vi "PicoScope4000aSetupStreaming.vi"(0 "error in":errorcluster, 2 "handle in":i16, 3 "Acquisition Settings":T2={"Auto Stop"=FALSE, "Desired Sample Interval"=4, "Pre-trigger Samples"=0, "Post-trigger Samples"=1000, "Down-Sample Ratio"=1, "Down-Sample Mode"=0, "Time Units"=2} {"Time Units" items=["Nanoseconds (ns)"=2, "Microseconds (us)"=3, "Milliseconds (ms)"=4, "Seconds (s)"=5]; "Down-Sample Mode" items=["None"=0, "Aggregate"=1, "Decimate"=2, "Average"=4]}, 4 "Buffer and Transfer Settings":T1={"startIndex"=0, "Samples"=1000000, "Down Sample Ratio"=1, "Down-Sample Mode"=0} {"Down-Sample Mode" items=["None"=0, "Aggregate"=1, "Decimate"=2, "Average"=4]; "Down Sample Ratio" step=1; "Samples" format="%_6p"}, 5 "enabled array":i16[](array[numeric]), 10 "Pointers In":u64[][](array[numeric])) -> (11 "Pointer array":u64[][](array[numeric]), 14 "error out":errorcluster, 16 "handle out":i16, 17 "Sample Interval":u32, 19 "sampleIntervalTimeUnits":u32)   [LabVIEW 2016]
doc: "Set up the data buffers and calls RunStreaming to start the device streaming.\nData will be copied from the driver buffers into the corresponding application buffers using the wrapper dll."
uses:
  ps4000a.dll
  ps4000aWrap.dll
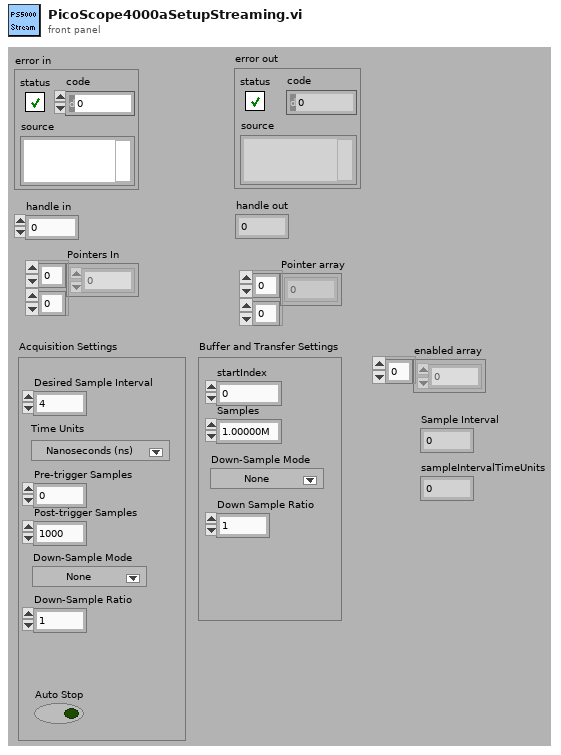
[diagram p1: front panel]
types:
  T1 = cluster{"startIndex":u64, "Samples":u64, "Down Sample Ratio":u64, "Down-Sample Mode":u32}
  T2 = cluster{"Auto Stop":bool, "Desired Sample Interval":u32, "Pre-trigger Samples":u32, "Post-trigger Samples":u32, "Down-Sample Ratio":u32, "Down-Sample Mode":i32, "Time Units":u32}
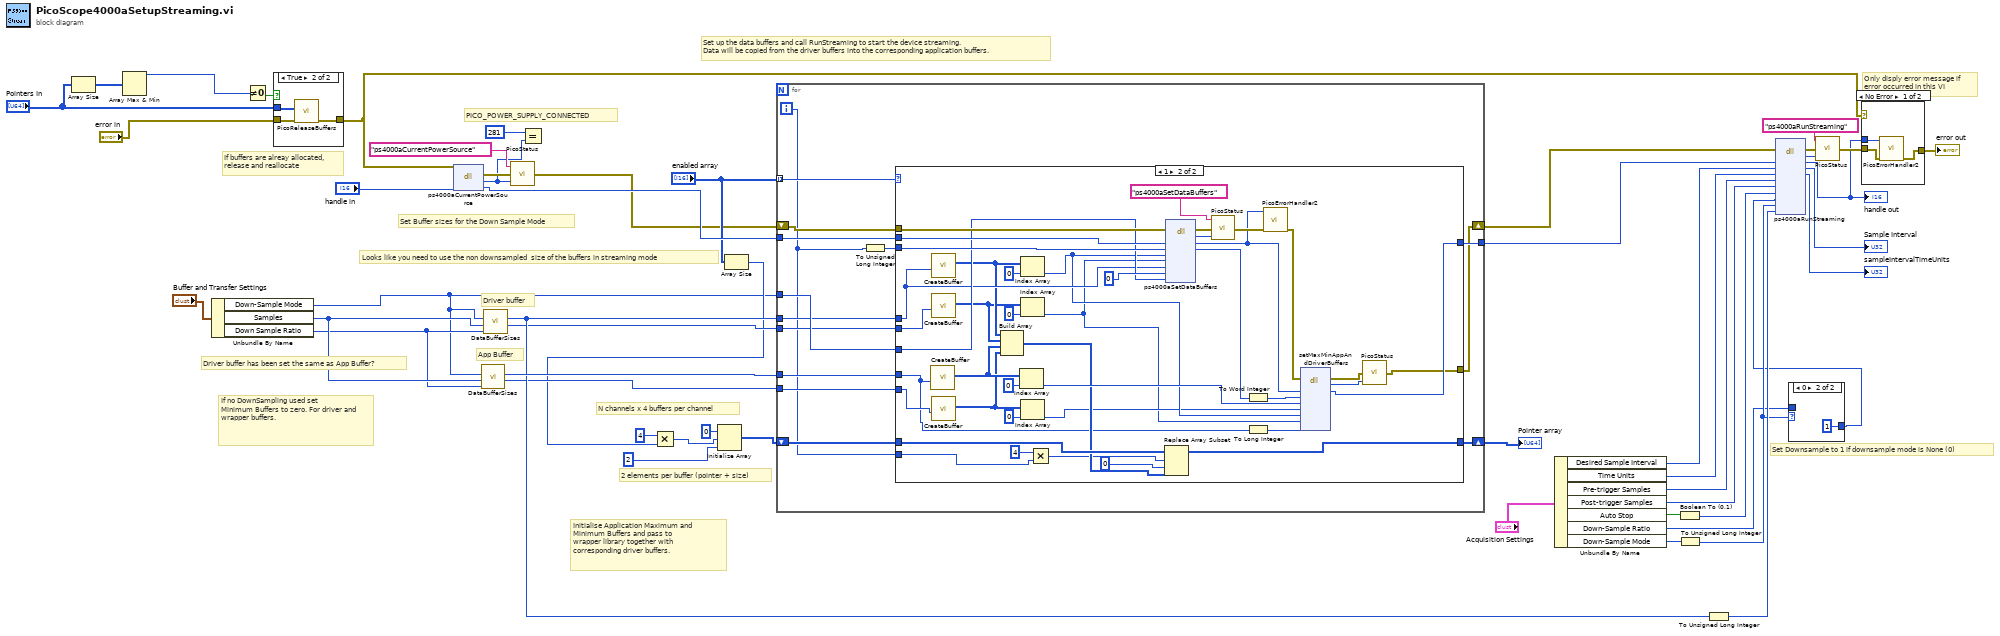
[diagram p0: block diagram]
diagram:
  # "Set Downsample to 1 if downsample mode is None (0)"
  # "Looks like you need to use the non downsampled  size of the buffers in streaming mode"
  # "If buffers are alreay allocated,\nrelease and reallocate"
  # "2 elements per buffer (pointer + size)"
  # "N channels x 4 buffers per channel"
  # "App Buffer"
  # "Driver buffer"
  # "Driver buffer has been set the same as App Buffer?"
  # "Set Buffer sizes for the Down Sample Mode"
  # "If no DownSampling used set \nMinimum Buffers to zero. For driver and wrapper buffers."
  # "PICO_POWER_SUPPLY_CONNECTED"
  # "Initialise Application Maximum and\nMinimum Buffers and pass to \nwrapper library together with corresponding driver buffers."
  # "Only disply error message if\nerror occurred in this VI"
  # "Set up the data buffers and call RunStreaming to start the device streaming.\nData will be copied from the driver buffers into the corresponding application buffers."
  n1 = Array Size(array="Pointers In") -> (size(s)=w7:i32[])
  n2 = Array Max & Min(array=w7) -> (max value=w6:i32)  [unwired: 3 out]
  n3 = Unbundle By Name("Buffer and Transfer Settings") -> ("Down-Sample Mode"=w4:u32, "Samples"=w30:u64, "Down Sample Ratio"=w29:u64)
  n4 = Not Equal To 0?(x=w6) -> (x != 0?=w14:bool)
  n5 = case shown="True" w14 {
    tunnel: "Pointers In" -> [_ w53]
    tunnel: "error in" -> [w52 w54]
    tunnel: [w52 w55] -> w11
    frame False {
    }
    frame True {
      n6 = call "PicoReleaseBuffers.vi"("error in (no error)"=w54, "Pointer array"=w53) -> ("error out"=w55:errorcluster)  [unwired: 9 in]
    }
  }
  n7 = dll-call lib="ps4000A.dll" fn="ps4000aCurrentPowerSource"(error in=w11, "handle"="handle in") -> (error out=w36:errorcluster, "PICO_STATUS"=w34:u32, "handle"=w33:i16)  [unwired: 2 in, 1 out]
  n8 = call "DataBufferSizes.vi"("Down Sample Ratio"=w29, "Number of Samples"=w30, "Down-Sample Mode"=w4) -> ("min Buffer Size"=w25:i32, "Max Buffer Size"=w28:i32)  [unwired: 7 in]
  n9 = call "DataBufferSizes.vi"("Down Sample Ratio"=w29, "Number of Samples"=w30, "Down-Sample Mode"=w4) -> ("min Buffer Size"=w26:i32, "Max Buffer Size"=w27:i32)  [unwired: 7 in]
  n10 = call "PicoStatus.vi"("PICO STATUS"=w34, "error in"=w36, "source"="ps4000aCurrentPowerSource") -> ("error out"=w10:errorcluster)
  n11 = Equal?(x=u32 281, y=w34) -> ()  [unwired: 1 out]
  n12 = Array Size(array="enabled array") -> (size(s)=w18:i32)
  n13 = Multiply(x=4, y=w18) -> (x*y=w19:i32)
  n14 = Initialize Array(u64 0 ("element"), w19, 2 ("dimension size")) -> (w8:u64[][])
  n15 = for {
    tunnel: "enabled array" -> [w61] mode=indexing
    tunnel: w33 -> [w69]
    tunnel: w4 -> [w68]
    tunnel: w28 -> [w67]
    tunnel: w27 -> [w66]
    tunnel: w26 -> [w65]
    tunnel: w25 -> [w64]
    tunnel: [w62] -> w21
    shift-right: [w60] -> w15
    shift-left: w10 -> [w59]
    shift-right: [w63] -> w24
    shift-left: w8 -> [w58]
    i -> [w56]
    n16 = To Unsigned Long Integer(number=w56) -> (unsigned 32bit integer=w57:u32)
    n17 = case shown="1" w61 {
      tunnel: w69 -> [w71 w113]
      tunnel: w59 -> [w70 w112]
      tunnel: w57 -> [_ w105]
      tunnel: w67 -> [_ w75]
      tunnel: w66 -> [_ w95]
      tunnel: w65 -> [_ w98]
      tunnel: w64 -> [_ w97]
      tunnel: w68 -> [_ w96]
      tunnel: w58 -> [w72 w89]
      tunnel: [w72 w88] -> w63
      tunnel: w56 -> [_ w85]
      tunnel: [w71 w81] -> w62
      tunnel: [w70 w80] -> w60
      frame 0, Default {
      }
      frame 1 {
        n18 = call "CreateBuffer.vi"("Buffer size"=w75) -> ("Pointer and BufferSize"=w91:u64[])  [unwired: 9 in, 1 out]
        n19 = call "CreateBuffer.vi"("Buffer size"=w95) -> ("Pointer and BufferSize"=w93:u64[])  [unwired: 9 in, 1 out]
        n20 = call "CreateBuffer.vi"("Buffer size"=w98) -> ("Pointer and BufferSize"=w92:u64[])  [unwired: 9 in, 1 out]
        n21 = call "CreateBuffer.vi"("Buffer size"=w97) -> ("Pointer and BufferSize"=w90:u64[])  [unwired: 9 in, 1 out]
        n22 = Build Array(w93, w92, w91, w90) -> (w84:u64[][])
        n23 = Index Array(array=w91, index=0) -> (element=w94:u64)
        n24 = Index Array(array=w93, index=0) -> (element=w87:u64)
        n25 = Index Array(array=w92, index=0) -> (element=w73:u64)
        n26 = Index Array(array=w90, index=0) -> (element=w74:u64)
        n27 = Multiply(x=4, y=w85) -> (x*y=w83:i32)
        n28 = Replace Array Subset(array=w89, new element=w84, index (row)=w83, index (col)=0 ("disabled index (row)")) -> (w88:u64[][])
        n29 = dll-call lib="ps4000a.dll" fn="ps4000aSetDataBuffers" ("ps3000.dll:_ps3000_open_unit@0")(error in=w112, "handle"=w113, "channel"=w105, "bufferMax"=w87, "bufferMin"=w73, "bufferLth"=w95, "segmentIndex"=u32 0, "downSampleRatioMode"=w96) -> (error out=w110:errorcluster, "PICO_STATUS"=w111:u32, "handle"=w77:i16, "channel"=w106:u32)  [unwired: 7 in, 1 out]
        n30 = call "PicoStatus.vi"("PICO STATUS"=w111, "error in"=w110, "source"="ps4000aSetDataBuffers") -> ("error out"=w79:errorcluster)
        n31 = To Word Integer(number=w106) -> (16bit integer=w107:i16)
        n32 = To Long Integer(number=w75) -> (32bit integer=w76:i32)
        n33 = call "PicoErrorHandler2.vi"("error in (no error)"=w79, "handle In"=w77) -> ("error out"=w78:errorcluster)  [unwired: 9 in]
        n34 = dll-call lib="ps4000aWrap.dll" fn="setMaxMinAppAndDriverBuffers"(error in=w78, "handle"=w77, "channel"=w107, "appMaxBuffer"=w94, "appMinBuffer"=w74, "driverMaxBuffer"=w87, "driverMinBuffer"=w73, "bufferLength"=w76) -> (error out=w104:errorcluster, "status"=w103:i16, "handle"=w81:i16)  [unwired: 8 in, 1 out]
        n35 = call "PicoStatus.vi"("PICO STATUS"=w103, "error in"=w104) -> ("error out"=w80:errorcluster)  [unwired: 1 in]
      }
    }
  }
  "Pointer array" <- w24
  n36 = Unbundle By Name("Acquisition Settings") -> ("Desired Sample Interval"=w44:u32, "Time Units"=w38:u32, "Pre-trigger Samples"=w43:u32, "Post-trigger Samples"=w42:u32, "Auto Stop"=w41:bool, "Down-Sample Ratio"=w2:u32, "Down-Sample Mode"=w39:i32)
  n37 = Boolean To (0,1)(Boolean=w41) -> (0, 1=w45:i16)
  n38 = To Unsigned Long Integer(number=w39) -> (unsigned 32bit integer=w3:u32)
  n39 = To Unsigned Long Integer(number=w27) -> (unsigned 32bit integer=w5:u32)
  n40 = case shown="0" w3 {
    tunnel: [w114 u32 1 ("Down-Sample Ratio")] -> w1
    tunnel: w2 -> [w114 _]
    frame Default {
    }
    frame 0 {
    }
  }
  n41 = dll-call lib="ps4000a.dll" fn="ps4000aRunStreaming" ("ps5000a.dll:_ps3000_open_unit@0")(error in=w15, "handle"=w21, "sampleInterval"=w44, "sampleIntervalTimeUnits"=w38, "maxPreTriggerSamples"=w43, "maxPostTriggerSamples"=w42, "autoStop"=w45, "downSampleRatio"=w1, "downSampleRatioMode"=w3, "overviewBufferSize"=w5) -> (error out=w49:errorcluster, "PICO_STATUS"=w50:u32, "handle"=w9:i16, "sampleInterval"=→"Sample Interval":u32, "sampleIntervalTimeUnits"=→"sampleIntervalTimeUnits":u32)  [unwired: 8 in, 1 out]
  "handle out" <- w9
  n42 = call "PicoStatus.vi"("PICO STATUS"=w50, "error in"=w49, "source"="ps4000aRunStreaming") -> ("error out"=w47:errorcluster)
  n43 = case shown="No Error" w11 {
    tunnel: [w117 w119] -> w51
    tunnel: w47 -> [w118 w119]
    tunnel: w9 -> [w116 _]
    frame No Error {
      n44 = call "PicoErrorHandler2.vi"("error in (no error)"=w118, "handle In"=w116) -> ("error out"=w117:errorcluster)  [unwired: 9 in]
    }
    frame Error {
    }
  }
  "error out" <- w51
